vi "Control-CaseFlow.vi"(0 "Camera Device  IN":T1, 1 "Image Device IN":cluster{"Image":T5, "errorImage":errorcluster}, 2 "DAQ Device IN":T3={"DAQ Fs (S/s)"=10000.0, "task"="", "error"={"status"=FALSE, "code"=0, "source"=""}, "Min Value"=-10.0, "Max Value"=10.0}, 3 "Time Control Parameters":cluster{"# samples":u32, "tiempos (ms)":dbl}, 4 "Parametros Maximos":T6, 5 "detla Parametros":T6, 6 "Camara ON?":bool, 7 "Control Parameters":T4={"N Init Avg"=6, "N Avg Best"=3, "% Best to test"=0.95, "% Best to beat"=1.0}, 8 "Control?":bool=TRUE, 9 "Reset Control":bool, 10 "Ajuste?":bool=TRUE, 11 "Calibracion DAQ":T2, 12 "Nueva Linea?":bool) -> (13 "Status Text":string, 14 "Camera Device OUT":T1, 15 "Image Device OUT":cluster{"Image":T5, "errorImage":errorcluster}, 16 "DAQ Device OUT":T3={"DAQ Fs (S/s)"=0.0, "task"="", "error"={"status"=FALSE, "code"=0, "source"=""}, "Min Value"=-10.0, "Max Value"=10.0}, 17 "Contraste":dbl, 18 "Waveform":waveform(dbl), 19 "Señal de Control":dbl[](array[numeric]))   [LabVIEW 2010]
uses:
  <vilib>/vision/Image Controls.llb/IMAQ Image.ctl
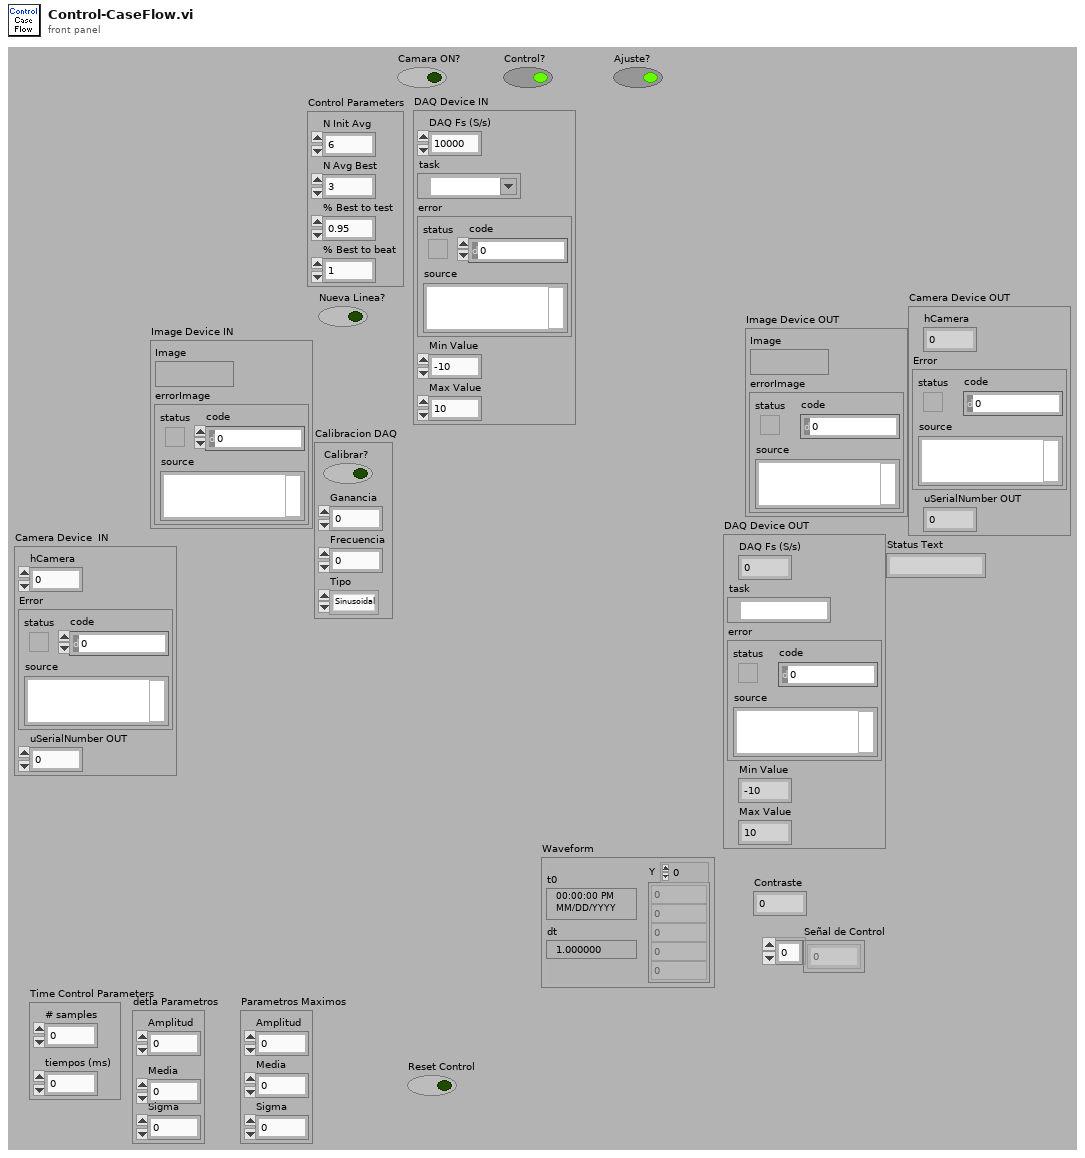
[diagram p1: front panel]
types:
  T1 = cluster{"hCamera":u32, "Error":errorcluster, "uSerialNumber OUT":u32}
  T2 = cluster{"Calibrar?":bool, "Ganancia":dbl, "Frecuencia":dbl, "Tipo":enum16{"Sinusoidal", "Triangular", "Cuadrada"}}
  T3 = cluster{"DAQ Fs (S/s)":dbl, "task":refnum<k21>, "error":errorcluster, "Min Value":dbl, "Max Value":dbl}
  T4 = cluster{"N Init Avg":u32, "N Avg Best":u32, "% Best to test":dbl, "% Best to beat":dbl}
  T5 = typedef "IMAQ Image.ctl" = refnum<image>
  T6 = cluster{"Amplitud":dbl, "Media":dbl, "Sigma":dbl}
  T7 = cluster{"DAQ Limits":cluster{"max":dbl, "min":dbl}, "Control Limits":cluster{"max":dbl, "min":dbl}}
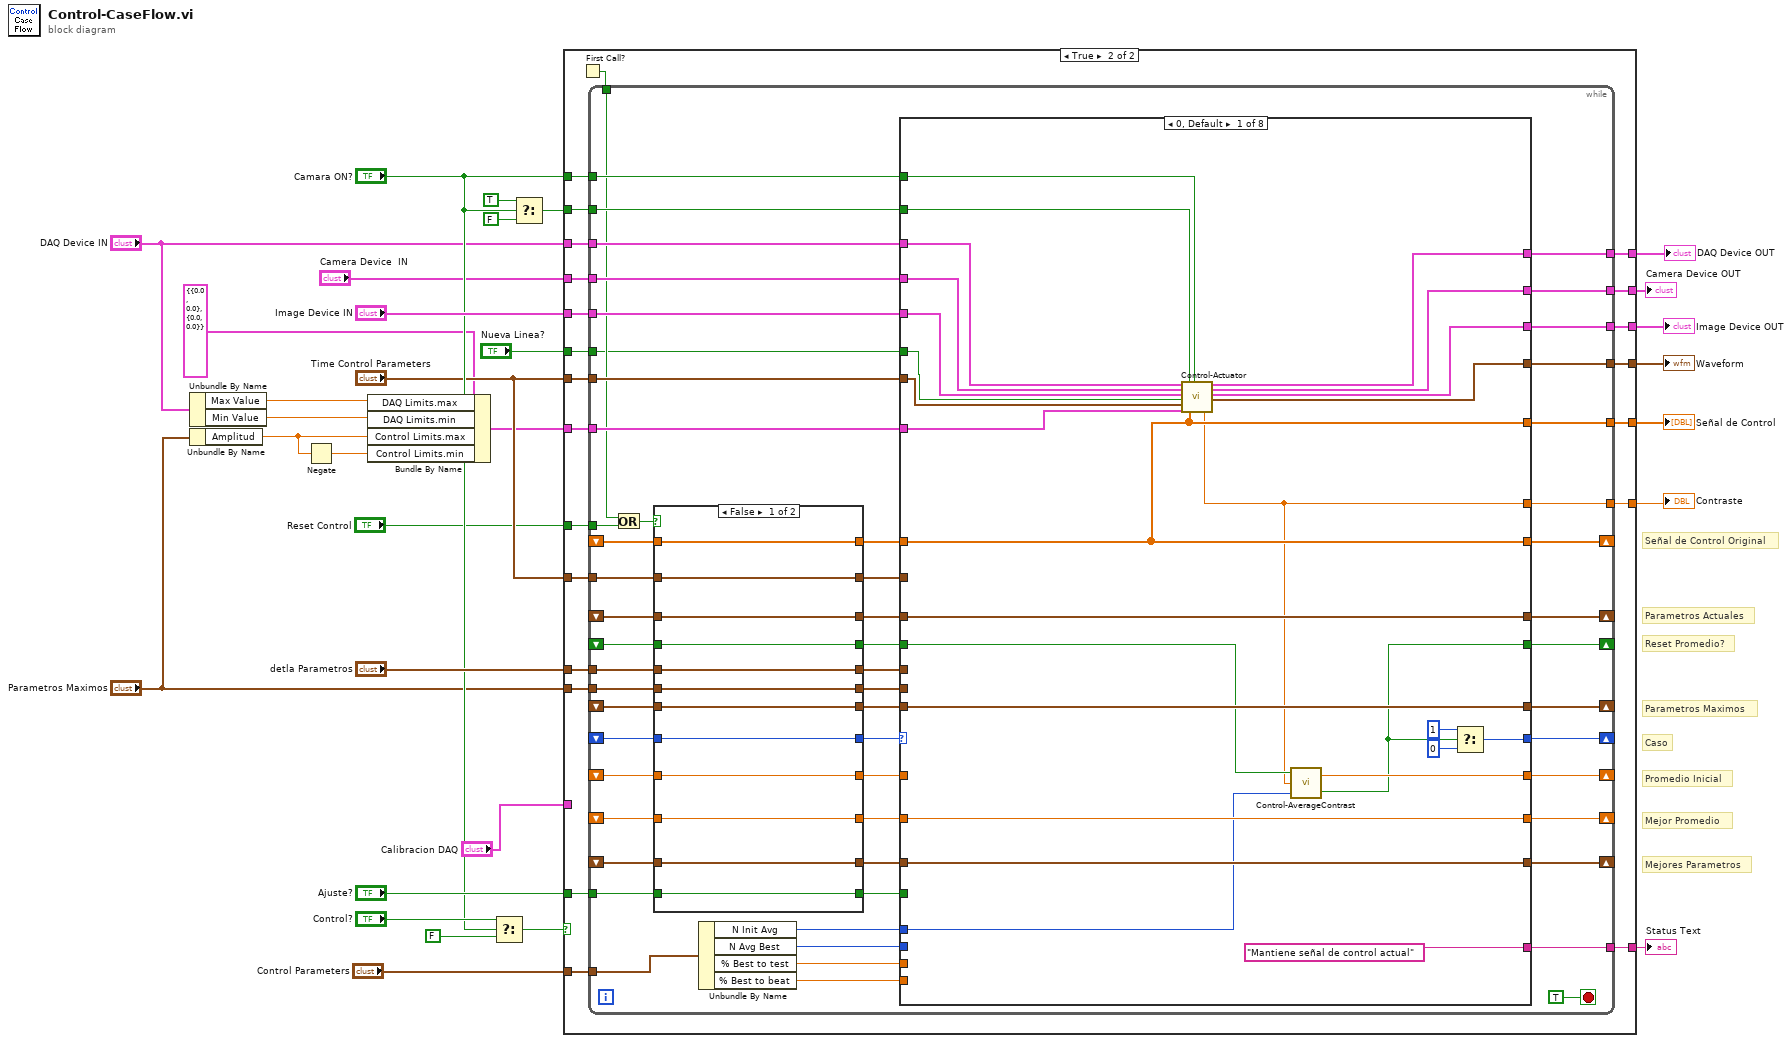
[diagram p0: block diagram]
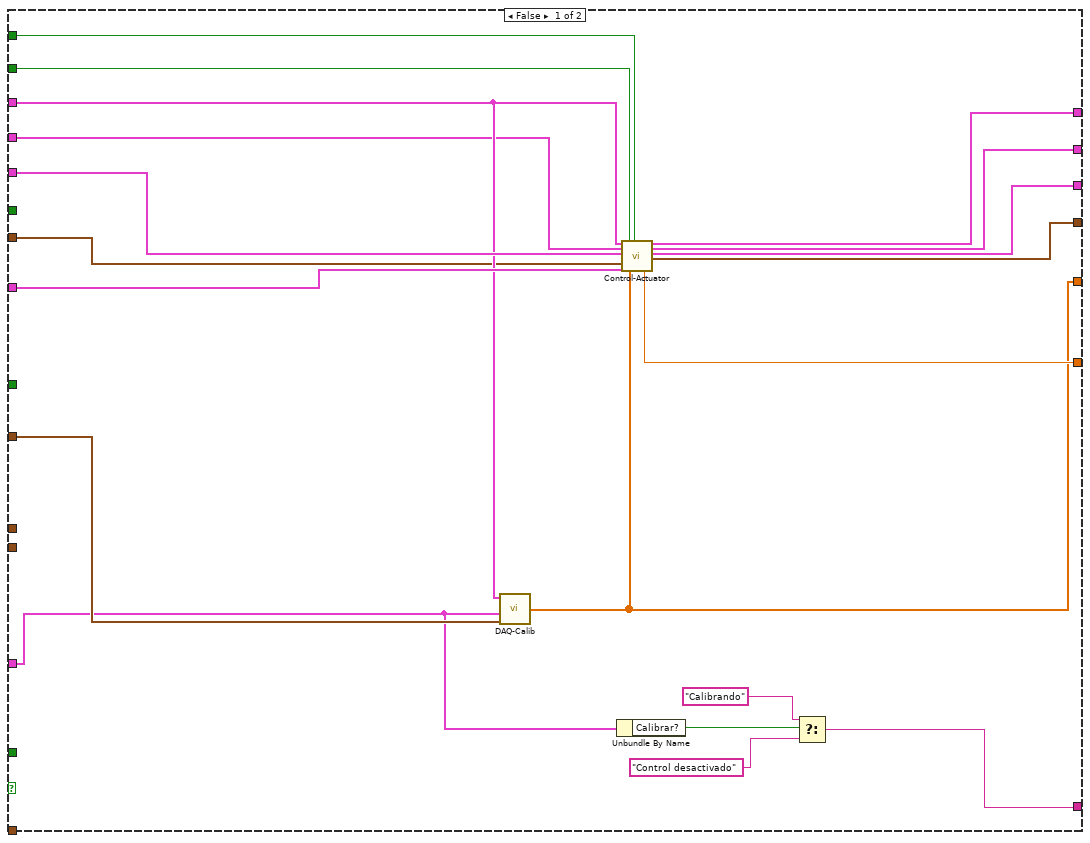
[diagram p2: hidden frame]
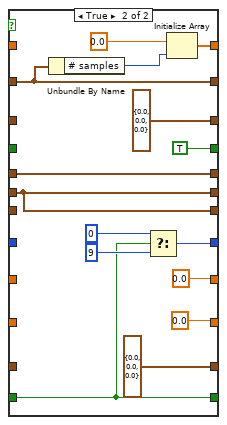
[diagram p3: hidden frame]
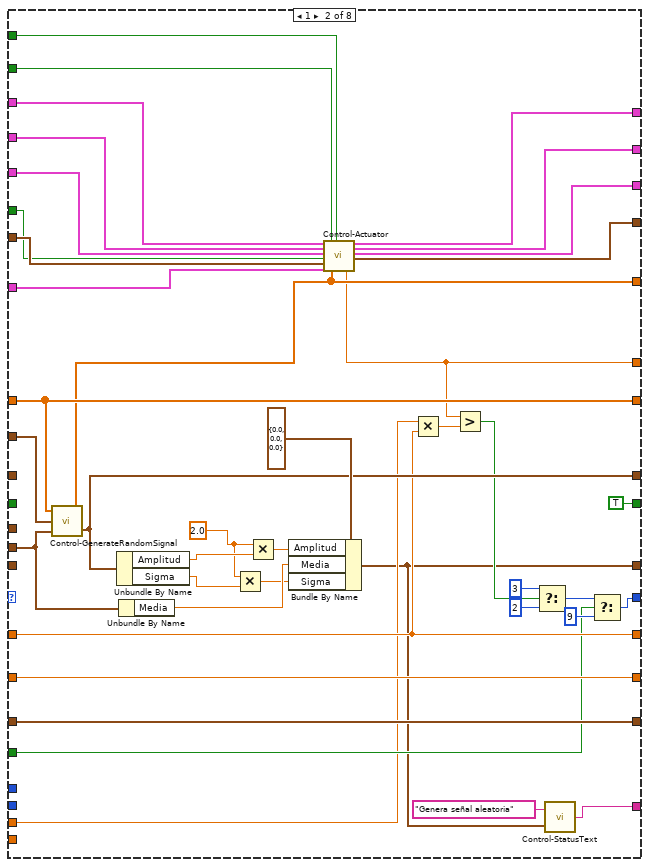
[diagram p4: hidden frame]
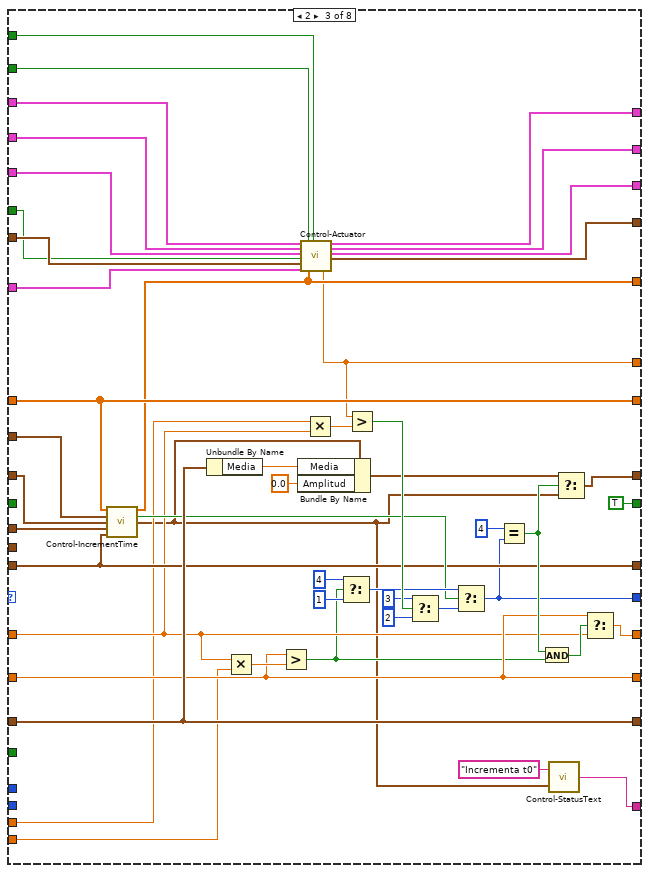
[diagram p5: hidden frame]
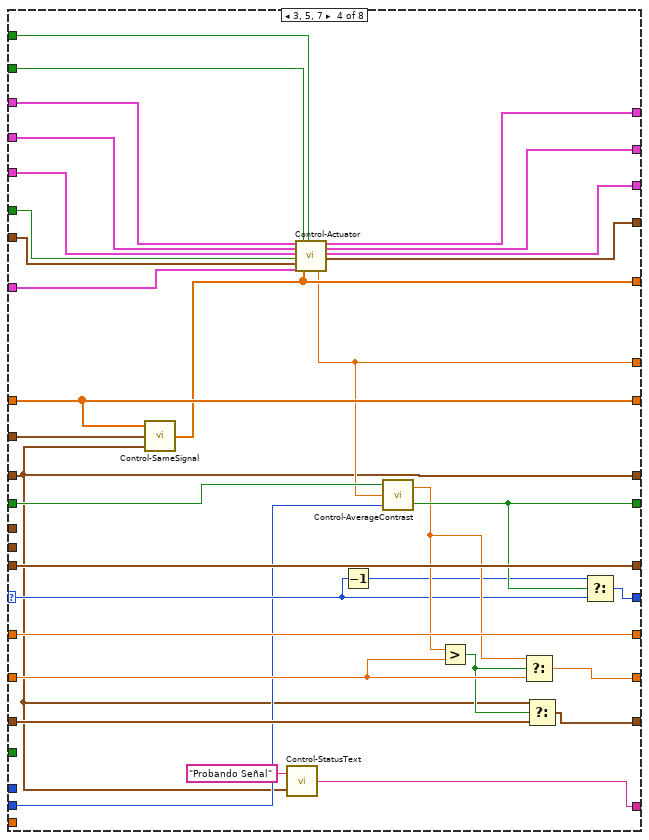
[diagram p6: hidden frame]
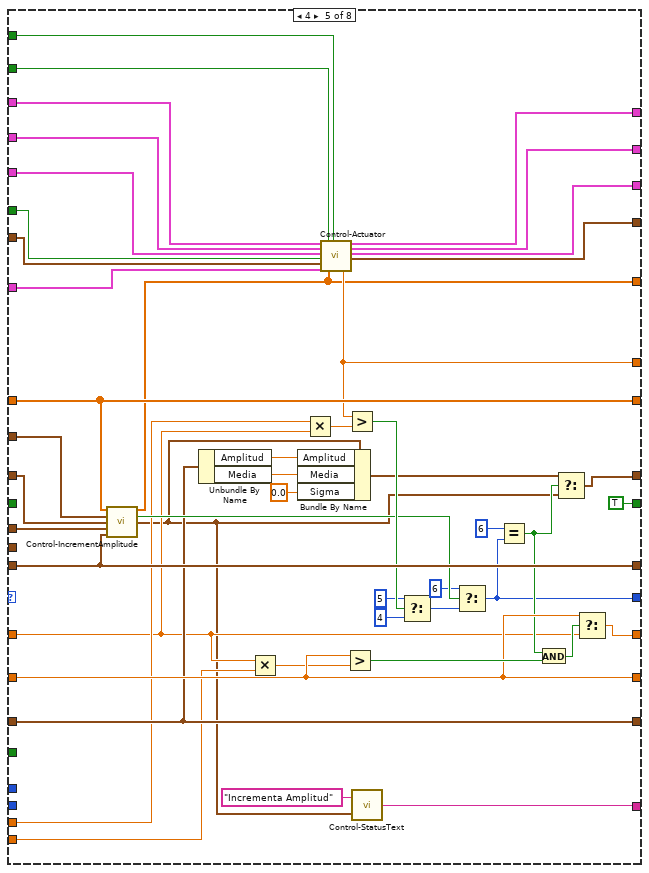
[diagram p7: hidden frame]
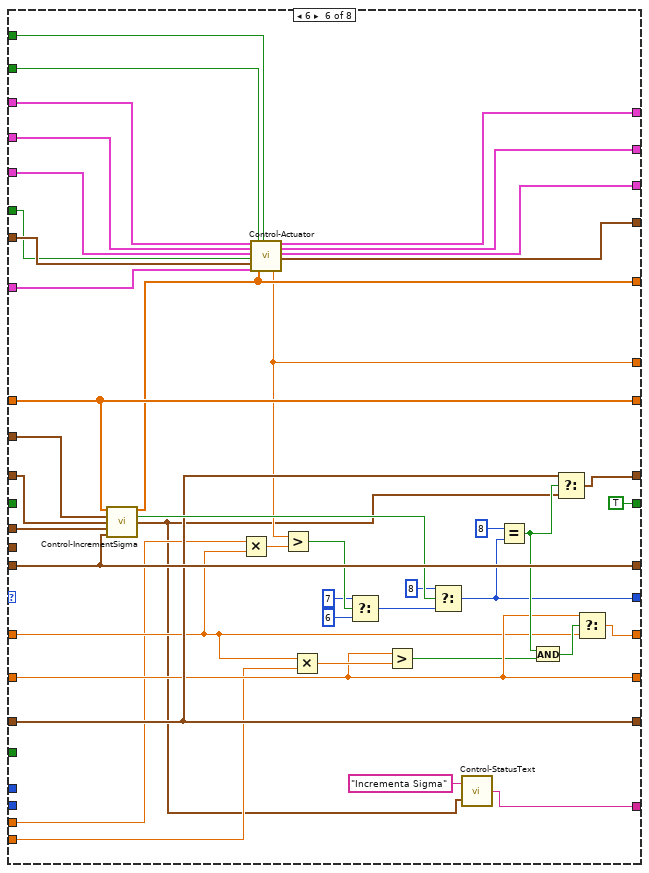
[diagram p8: hidden frame]
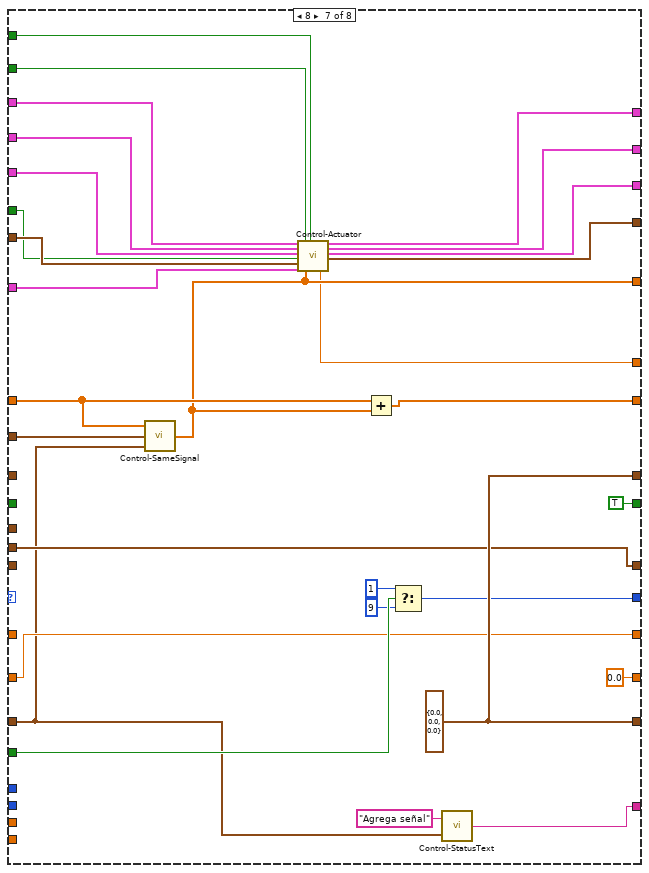
[diagram p9: hidden frame]
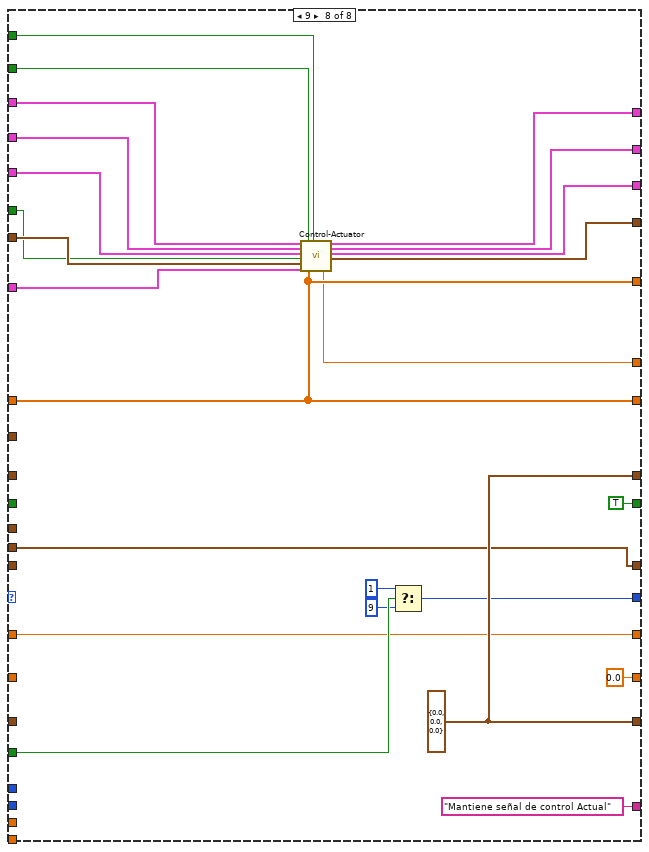
[diagram p10: hidden frame]
diagram:
  # "Reset Promedio?"
  # "Mejores Parametros"
  # "Mejor Promedio"
  # "Señal de Control Original"
  # "Parametros Actuales"
  # "Parametros Maximos"
  # "Caso"
  # "Promedio Inicial"
  n1 = Unbundle By Name("DAQ Device IN") -> ("Max Value"=w11:dbl, "Min Value"=w10:dbl)
  n2 = Unbundle By Name("Parametros Maximos") -> ("Amplitud"=w8:dbl)
  n3 = Negate(x=w8) -> (-x=w9:dbl)
  n4 = Bundle By Name(cluster=T7 {"DAQ Limits"={"max"=0.0, "min"=0.0}, "Control Limits"={"max"=0.0, "min"=0.0}} ("Limites"), "DAQ Limits.max"=w11, "DAQ Limits.min"=w10, "Control Limits.max"=w8, "Control Limits.min"=w9) -> (w12:T7)
  n5 = Select(t="Control?", s="Camara ON?", f=FALSE) -> (s? t:f=w21:bool)
  n6 = Select(t=TRUE, s="Camara ON?", f=FALSE) -> (s? t:f=w24:bool)
  n7 = case shown="True" w21 {
    tunnel: "Time Control Parameters" -> [w38 w72]
    tunnel: "detla Parametros" -> [_ w71]
    tunnel: "Parametros Maximos" -> [_ w70]
    tunnel: "Ajuste?" -> [_ w68]
    tunnel: [w40 w67] -> w29
    tunnel: [w50 w66] -> w28
    tunnel: w12 -> [w49 w65]
    tunnel: "Time Control Parameters" -> [w37 w64]
    tunnel: "Image Device IN" -> [w48 w63]
    tunnel: "Camera Device  IN" -> [w39 w62]
    tunnel: "DAQ Device IN" -> [w41 w61]
    tunnel: w24 -> [w47 w60]
    tunnel: "Camara ON?" -> [w46 w59]
    tunnel: [w45 w58] -> w26
    tunnel: [w44 w57] -> w25
    tunnel: [w43 w56] -> w3
    tunnel: [w42 w55] -> w14
    tunnel: "Reset Control" -> [_ w54]
    tunnel: "Control Parameters" -> [_ w53]
    tunnel: "Calibracion DAQ" -> [w33 _]
    tunnel: [w32 w52] -> w2
    tunnel: "Nueva Linea?" -> [_ w51]
    frame False {
      n8 = call "DAQ-Calib.vi"("Time Control Parameters"=w38, "Calibracion DAQ"=w33, "DAQ Device IN"=w41) -> ("Calibration OUT"=w40:dbl[])  [unwired: 1 in]
      n9 = Unbundle By Name(w33) -> ("Calibrar?"=w36:bool)
      n10 = call "Control-Actuator.vi"("DAQ Device IN"=w41, "Camera Device  IN"=w39, "Image Device IN"=w48, "Time Control Parameters"=w37, "Limites"=w49, "DAQ?"=w47, "ControlSignal"=w40, "Streeam?"=w46) -> ("Contraste"=w50:dbl, "DAQ Device OUT"=w42:T3, "Camera Device OUT"=w43:T1, "Image Device OUT"=w44:cluster{"Image":T5, "errorImage":errorcluster}, "Waveform"=w45:waveform(dbl))  [unwired: 7 in]
      n11 = Select(t="Calibrando", s=w36, f="Control desactivado") -> (s? t:f=w32:string)
    }
    frame True {
      n12 = First Call?() -> (First Call?: T/F=w69:bool)
      n13 = while {
        shift-right: [w125] -> _
        shift-left: _ -> [w112]
        tunnel: w72 -> [w104]
        shift-right: [w128] -> _
        shift-left: _ -> [w120]
        shift-right: [w127] -> _
        shift-left: _ -> [w114]
        shift-right: [w126] -> _
        shift-left: _ -> [w118]
        shift-right: [w124] -> _
        shift-left: _ -> [w110]
        tunnel: w71 -> [w101]
        shift-right: [w123] -> _
        shift-left: _ -> [w108]
        shift-right: [w122] -> _
        shift-left: _ -> [w106]
        shift-right: [w121] -> _
        shift-left: _ -> [w116]
        tunnel: w68 -> [w103]
        tunnel: w70 -> [w102]
        tunnel: w69 -> [w82]
        tunnel: [w96] -> w67
        tunnel: [w95] -> w66
        tunnel: w65 -> [w94]
        tunnel: w64 -> [w93]
        tunnel: w63 -> [w92]
        tunnel: w62 -> [w91]
        tunnel: w61 -> [w90]
        tunnel: w60 -> [w89]
        tunnel: w59 -> [w88]
        tunnel: [w87] -> w58
        tunnel: [w86] -> w57
        tunnel: [w85] -> w56
        tunnel: [w84] -> w55
        tunnel: w54 -> [w80]
        tunnel: w53 -> [w79]
        tunnel: [w74] -> w52
        tunnel: w51 -> [w73]
        stop <- TRUE stop-if-true
        n14 = Or(x=w82, y=w80) -> (x .or. y?=w81:bool)
        n15 = case shown="False" w81 {
          tunnel: w120 -> [w140 _]
          tunnel: [w140 w155] -> w119
          tunnel: [w139 T6 {"Amplitud"=0.0, "Media"=0.0, "Sigma"=0.0} ("Parametros Iniciales")] -> w117
          tunnel: w118 -> [w139 _]
          tunnel: w116 -> [w138 _]
          tunnel: [w138 TRUE] -> w115
          tunnel: w114 -> [w137 _]
          tunnel: [w137 w144] -> w113
          tunnel: w112 -> [w136 _]
          tunnel: [w136 w145] -> w111
          tunnel: w110 -> [w135 _]
          tunnel: [w135 0.0 ("Contraste Promedio")] -> w109
          tunnel: w108 -> [w134 _]
          tunnel: [w134 0.0 ("Contraste Promedio")] -> w107
          tunnel: w106 -> [w133 _]
          tunnel: [w133 T6 {"Amplitud"=0.0, "Media"=0.0, "Sigma"=0.0} ("Parametros Maximos")] -> w105
          tunnel: w104 -> [w132 w141]
          tunnel: w102 -> [w130 w144]
          tunnel: w103 -> [w129 w142]
          tunnel: [w130 w144] -> w100
          tunnel: [w131 w143] -> w99
          tunnel: w101 -> [w131 w143]
          tunnel: [w129 w142] -> w98
          tunnel: [w132 w141] -> w97
          frame False {
          }
          frame True {
            n16 = Unbundle By Name(w141) -> ("# samples"=w153:u32)
            n17 = Select(t=u32 0, s=w142, f=u32 9) -> (s? t:f=w145:u32)
            n18 = Initialize Array(0.0 ("element"), w153) -> (w155:dbl[])
          }
        }
        n19 = Unbundle By Name(w79) -> ("N Init Avg"=w78:u32, "N Avg Best"=w77:u32, "% Best to test"=w76:dbl, "% Best to beat"=w75:dbl)
        n20 = case shown="0, Default" w111 {
          selector: w111 -> [_ _ _ w289 _ _ _ _]
          tunnel: w119 -> [w171 w221 w267 w302 w347 w390 w415 w437]
          tunnel: w97 -> [_ w222 w270 w303 w350 w393 w422 _]
          tunnel: w113 -> [w174 _ w251 w294 w346 w389 _ _]
          tunnel: [w171 w221 w267 w302 w347 w390 w414 w437] -> w128
          tunnel: [w174 w183 w251 w294 w346 w389 w411 w439] -> w127
          tunnel: [w175 w219 w257 w273 w336 w381 w420 w445] -> w126
          tunnel: [w181 w189 w235 w301 w315 w361 w412 w440] -> w125
          tunnel: [w176 w211 w261 w300 w341 w385 w413 w438] -> w124
          tunnel: w109 -> [_ w211 w230 w300 w308 w357 _ w438]
          tunnel: [w170 w190 w249 w287 w328 w376 w409 w436] -> w95
          tunnel: [w171 w205 w250 w288 w327 w377 w410 w437] -> w96
          tunnel: w117 -> [w175 _ w269 w273 w349 w392 _ _]
          tunnel: w99 -> [_ _ w268 _ w348 w391 _ _]
          tunnel: [w177 w214 w232 w299 w339 w359 0.0 ("Contraste Promedio") 0.0 ("Contraste Promedio")] -> w123
          tunnel: [w178 w213 w255 w297 w334 w378 w420 w445] -> w122
          tunnel: w105 -> [w178 w213 w255 w295 w334 w378 w395 _]
          tunnel: w107 -> [w177 w214 w232 w298 w339 w359 w413 _]
          tunnel: w115 -> [w172 _ _ w293 _ _ _ _]
          tunnel: [w173 TRUE ("Llego a N?") TRUE ("Llego a N?") w292 TRUE ("Llego a N?") TRUE ("Llego a N?") TRUE ("Llego a N?") TRUE ("Llego a N?")] -> w121
          tunnel: w98 -> [_ w191 _ _ _ _ w418 w443]
          tunnel: w100 -> [_ w206 _ _ _ _ w411 w439]
          tunnel: w94 -> [w169 w204 w248 w286 w312 w375 w408 w435]
          tunnel: w93 -> [w168 w203 w247 w285 w313 w372 w407 w434]
          tunnel: w92 -> [w167 w202 w246 w284 w326 w371 w406 w433]
          tunnel: w91 -> [w166 w201 w245 w283 w325 w370 w405 w432]
          tunnel: w90 -> [w165 w194 w244 w282 w314 w369 w404 w431]
          tunnel: w89 -> [w164 w200 w243 w281 w324 w373 w403 w430]
          tunnel: w88 -> [w163 w199 w242 w280 w323 w374 w402 w429]
          tunnel: [w162 w198 w241 w279 w322 w368 w401 w428] -> w87
          tunnel: [w161 w196 w240 w278 w321 w367 w400 w427] -> w86
          tunnel: [w160 w197 w239 w277 w320 w366 w399 w426] -> w85
          tunnel: [w159 w195 w238 w276 w319 w365 w398 w425] -> w84
          tunnel: w78 -> [w158 _ _ _ _ _ _ _]
          tunnel: w77 -> [_ _ _ w275 _ _ _ _]
          tunnel: w76 -> [_ w188 w228 _ w311 w356 _ _]
          tunnel: w75 -> [_ _ w231 _ w310 w358 _ _]
          tunnel: ["Mantiene señal de control actual" w185 w226 w274 w307 w354 w397 "Mantiene señal de control Actual"] -> w74
          tunnel: w73 -> [w156 w182 w223 w271 w304 w351 w394 w423]
          frame 0, Default {
            n21 = call "Control-Actuator.vi"("DAQ Device IN"=w165, "Camera Device  IN"=w166, "Image Device IN"=w167, "Nueva Linea?"=w156, "Time Control Parameters"=w168, "Limites"=w169, "DAQ?"=w164, "ControlSignal"=w171, "Streeam?"=w163) -> ("Contraste"=w170:dbl, "DAQ Device OUT"=w159:T3, "Camera Device OUT"=w160:T1, "Image Device OUT"=w161:cluster{"Image":T5, "errorImage":errorcluster}, "Waveform"=w162:waveform(dbl))  [unwired: 6 in]
            n22 = call "Control-AverageContrast.vi"("N"=w158, "Contraste"=w170, "Reset"=w172) -> ("Llego a N?"=w173:bool, "Contraste Promedio"=w176:dbl)
            n23 = Select(t=u32 1, s=w173, f=u32 0) -> (s? t:f=w181:u32)
          }
          frame 1 {
            w215 = 2.0 ("x")
            n24 = call "Control-GenerateRandomSignal.vi"("Parametros Maximos"=w206, "Sound Parameters"=w222, "Señal de Control IN"=w221) -> ("Parametros Iniciales"=w219:T6, "Out"=w205:dbl[])
            n25 = Unbundle By Name(w219) -> ("Amplitud"=w218:dbl, "Sigma"=w216:dbl)
            n26 = Unbundle By Name(w206) -> ("Media"=w217:dbl)
            n27 = Multiply(x=w215, y=w216) -> (x*y=w186:dbl)
            n28 = Multiply(x=w215, y=w218) -> (x*y=w187:dbl)
            n29 = Bundle By Name(cluster=T6 {"Amplitud"=0.0, "Media"=0.0, "Sigma"=0.0} ("Parametros Iniciales"), "Amplitud"=w187, "Media"=w217, "Sigma"=w186) -> (w183:T6)
            n30 = call "Control-Actuator.vi"("DAQ Device IN"=w194, "Camera Device  IN"=w201, "Image Device IN"=w202, "Nueva Linea?"=w182, "Time Control Parameters"=w203, "Limites"=w204, "DAQ?"=w200, "ControlSignal"=w205, "Streeam?"=w199) -> ("Contraste"=w190:dbl, "DAQ Device OUT"=w195:T3, "Camera Device OUT"=w197:T1, "Image Device OUT"=w196:cluster{"Image":T5, "errorImage":errorcluster}, "Waveform"=w198:waveform(dbl))  [unwired: 6 in]
            n31 = Multiply(x=w188, y=w211) -> (x*y=w212:dbl)
            n32 = Greater?(x=w190, y=w212) -> (0:w210:bool)
            n33 = Select(t=u32 3, s=w210, f=u32 2) -> (s? t:f=w192:u32)
            n34 = call "Control-StatusText.vi"("Parametros Actuales"=w183, "string"="Genera señal aleatoria") -> ("String"=w185:string)
            n35 = Select(t=w192, s=w191, f=u32 9) -> (s? t:f=w189:u32)
          }
          frame 2 {
            n36 = call "Control-IncrementTime.vi"("Señal de Control IN"=w267, "Sound Parameters"=w270, "Parametros Actuales IN"=w269, "detla Parametros"=w268, "Parametros Maximos"=w251) -> ("Out"=w250:dbl[], "Tope?"=w253:bool, "Parametros Actuales OUT"=w225:T6)  [unwired: 8 in]
            n37 = Unbundle By Name(w255) -> ("Media"=w227:dbl)
            n38 = Multiply(x=w230, y=w231) -> (x*y=w233:dbl)
            n39 = Greater?(x=w232, y=w233) -> (0:w229:bool)
            n40 = Bundle By Name(cluster=w225, "Media"=w227, "Amplitud"=0.0) -> (w256:T6)
            n41 = call "Control-Actuator.vi"("DAQ Device IN"=w244, "Camera Device  IN"=w245, "Image Device IN"=w246, "Nueva Linea?"=w223, "Time Control Parameters"=w247, "Limites"=w248, "DAQ?"=w243, "ControlSignal"=w250, "Streeam?"=w242) -> ("Contraste"=w249:dbl, "DAQ Device OUT"=w238:T3, "Camera Device OUT"=w239:T1, "Image Device OUT"=w240:cluster{"Image":T5, "errorImage":errorcluster}, "Waveform"=w241:waveform(dbl))  [unwired: 6 in]
            n42 = Multiply(x=w228, y=w230) -> (x*y=w266:dbl)
            n43 = Select(t=u32 4, s=w229, f=u32 1) -> (s? t:f=w262:u32)
            n44 = Greater?(x=w249, y=w266) -> (0:w265:bool)
            n45 = Select(t=u32 3, s=w265, f=u32 2) -> (s? t:f=w234:u32)
            n46 = Select(t=w262, s=w253, f=w234) -> (s? t:f=w235:u32)
            n47 = Equal?(x=u32 4, y=w235) -> (x = y?=w252:bool)
            n48 = And(x=w252, y=w229) -> (x .and. y?=w260:bool)
            n49 = call "Control-StatusText.vi"("Parametros Actuales"=w225, "string"="Incrementa t0") -> ("String"=w226:string)
            n50 = Select(t=w256, s=w252, f=w225) -> (s? t:f=w257:T6)
            n51 = Select(t=w232, s=w260, f=w230) -> (s? t:f=w261:dbl)
          }
          frame 3, 5, 7 {
            n52 = call "Control-SameSignal.vi"("Parametros Actuales IN"=w273, "Sound Parameters"=w303, "Señal de Control IN"=w302) -> ("Out"=w288:dbl[])
            n53 = call "Control-StatusText.vi"("Parametros Actuales"=w273, "string"="Probando Señal") -> ("String"=w274:string)
            n54 = call "Control-Actuator.vi"("DAQ Device IN"=w282, "Camera Device  IN"=w283, "Image Device IN"=w284, "Nueva Linea?"=w271, "Time Control Parameters"=w285, "Limites"=w286, "DAQ?"=w281, "ControlSignal"=w288, "Streeam?"=w280) -> ("Contraste"=w287:dbl, "DAQ Device OUT"=w276:T3, "Camera Device OUT"=w277:T1, "Image Device OUT"=w278:cluster{"Image":T5, "errorImage":errorcluster}, "Waveform"=w279:waveform(dbl))  [unwired: 6 in]
            n55 = Decrement(x=w289) -> (x-1=w290:u32)
            n56 = call "Control-AverageContrast.vi"("N"=w275, "Contraste"=w287, "Reset"=w293) -> ("Llego a N?"=w292:bool, "Contraste Promedio"=w291:dbl)
            n57 = Greater?(x=w291, y=w298) -> (0:w296:bool)
            n58 = Select(t=w291, s=w296, f=w298) -> (s? t:f=w299:dbl)
            n59 = Select(t=w273, s=w296, f=w295) -> (s? t:f=w297:T6)
            n60 = Select(t=w290, s=w292, f=w289) -> (s? t:f=w301:u32)
          }
          frame 4 {
            n61 = call "Control-IncrementAmplitude.vi"("Señal de Control IN"=w347, "Sound Parameters"=w350, "Parametros Actuales IN"=w349, "detla Parametros"=w348, "Parametros Maximos"=w346) -> ("Out"=w327:dbl[], "Tope?"=w343:bool, "Parametros Actuales OUT"=w305:T6)  [unwired: 8 in]
            n62 = Unbundle By Name(w334) -> ("Amplitud"=w333:dbl, "Media"=w331:dbl)
            n63 = Multiply(x=w308, y=w310) -> (x*y=w309:dbl)
            n64 = Bundle By Name(cluster=w305, "Amplitud"=w333, "Media"=w331, "Sigma"=0.0 ("Amplitud")) -> (w335:T6)
            n65 = Multiply(x=w311, y=w308) -> (x*y=w345:dbl)
            n66 = call "Control-Actuator.vi"("DAQ Device IN"=w314, "Camera Device  IN"=w325, "Image Device IN"=w326, "Nueva Linea?"=w304, "Time Control Parameters"=w313, "Limites"=w312, "DAQ?"=w324, "ControlSignal"=w327, "Streeam?"=w323) -> ("Contraste"=w328:dbl, "DAQ Device OUT"=w319:T3, "Camera Device OUT"=w320:T1, "Image Device OUT"=w321:cluster{"Image":T5, "errorImage":errorcluster}, "Waveform"=w322:waveform(dbl))  [unwired: 6 in]
            n67 = Greater?(x=w339, y=w309) -> (0:w342:bool)
            n68 = Greater?(x=w328, y=w345) -> (0:w344:bool)
            n69 = call "Control-StatusText.vi"("Parametros Actuales"=w305, "string"="Incrementa Amplitud") -> ("String"=w307:string)
            n70 = Select(t=u32 5, s=w344, f=u32 4) -> (s? t:f=w316:u32)
            n71 = Select(t=u32 6, s=w343, f=w316) -> (s? t:f=w315:u32)
            n72 = Equal?(x=u32 6, y=w315) -> (x = y?=w329:bool)
            n73 = And(x=w329, y=w342) -> (x .and. y?=w340:bool)
            n74 = Select(t=w335, s=w329, f=w305) -> (s? t:f=w336:T6)
            n75 = Select(t=w339, s=w340, f=w308) -> (s? t:f=w341:dbl)
          }
          frame 6 {
            n76 = call "Control-IncrementSigma.vi"("Señal de Control IN"=w390, "Sound Parameters"=w393, "Parametros Actuales IN"=w392, "detla Parametros"=w391, "Parametros Maximos"=w389) -> ("Out"=w377:dbl[], "Tope?"=w386:bool, "Parametros Actuales OUT"=w353:T6)  [unwired: 8 in]
            n77 = Multiply(x=w356, y=w357) -> (x*y=w388:dbl)
            n78 = call "Control-Actuator.vi"("DAQ Device IN"=w369, "Camera Device  IN"=w370, "Image Device IN"=w371, "Nueva Linea?"=w351, "Time Control Parameters"=w372, "Limites"=w375, "DAQ?"=w373, "ControlSignal"=w377, "Streeam?"=w374) -> ("Contraste"=w376:dbl, "DAQ Device OUT"=w365:T3, "Camera Device OUT"=w366:T1, "Image Device OUT"=w367:cluster{"Image":T5, "errorImage":errorcluster}, "Waveform"=w368:waveform(dbl))  [unwired: 6 in]
            n79 = Greater?(x=w376, y=w388) -> (0:w387:bool)
            n80 = Multiply(x=w357, y=w358) -> (x*y=w360:dbl)
            n81 = Select(t=u32 7, s=w387, f=u32 6) -> (s? t:f=w362:u32)
            n82 = Greater?(x=w359, y=w360) -> (0:w355:bool)
            n83 = Select(t=u32 8, s=w386, f=w362) -> (s? t:f=w361:u32)
            n84 = call "Control-StatusText.vi"("Parametros Actuales"=w353, "string"="Incrementa Sigma") -> ("String"=w354:string)
            n85 = Equal?(x=u32 8, y=w361) -> (x = y?=w379:bool)
            n86 = And(x=w379, y=w355) -> (x .and. y?=w384:bool)
            n87 = Select(t=w378, s=w379, f=w353) -> (s? t:f=w381:T6)
            n88 = Select(t=w359, s=w384, f=w357) -> (s? t:f=w385:dbl)
          }
          frame 8 {
            w420 = T6 {"Amplitud"=0.0, "Media"=0.0, "Sigma"=0.0} ("Parametros Maximos")
            n89 = call "Control-SameSignal.vi"("Parametros Actuales IN"=w395, "Sound Parameters"=w422, "Señal de Control IN"=w415) -> ("Out"=w410:dbl[])
            n90 = call "Control-Actuator.vi"("DAQ Device IN"=w404, "Camera Device  IN"=w405, "Image Device IN"=w406, "Nueva Linea?"=w394, "Time Control Parameters"=w407, "Limites"=w408, "DAQ?"=w403, "ControlSignal"=w410, "Streeam?"=w402) -> ("Contraste"=w409:dbl, "DAQ Device OUT"=w398:T3, "Camera Device OUT"=w399:T1, "Image Device OUT"=w400:cluster{"Image":T5, "errorImage":errorcluster}, "Waveform"=w401:waveform(dbl))  [unwired: 6 in]
            n91 = Add(x=w415, y=w410) -> (x+y=w414:dbl[])
            n92 = Select(t=u32 1, s=w418, f=u32 9) -> (s? t:f=w412:u32)
            n93 = call "Control-StatusText.vi"("Parametros Actuales"=w395, "string"="Agrega señal") -> ("String"=w397:string)
          }
          frame 9 {
            w445 = T6 {"Amplitud"=0.0, "Media"=0.0, "Sigma"=0.0} ("Parametros Maximos")
            n94 = call "Control-Actuator.vi"("DAQ Device IN"=w431, "Camera Device  IN"=w432, "Image Device IN"=w433, "Nueva Linea?"=w423, "Time Control Parameters"=w434, "Limites"=w435, "DAQ?"=w430, "ControlSignal"=w437, "Streeam?"=w429) -> ("Contraste"=w436:dbl, "DAQ Device OUT"=w425:T3, "Camera Device OUT"=w426:T1, "Image Device OUT"=w427:cluster{"Image":T5, "errorImage":errorcluster}, "Waveform"=w428:waveform(dbl))  [unwired: 6 in]
            n95 = Select(t=u32 1, s=w443, f=u32 9) -> (s? t:f=w440:u32)
          }
        }
      }
    }
  }
  "Señal de Control" <- w29
  "Contraste" <- w28
  "Image Device OUT" <- w25
  "Waveform" <- w26
  "DAQ Device OUT" <- w14
  "Camera Device OUT" <- w3
  "Status Text" <- w2
